vi "Test App Removing Process Triggers Broadcast.vi"(8 "error in (no error)":errorcluster, 11 "Rig Test in":refnum<class "Application Test.lvclass">) -> (0 "error out":errorcluster, 3 "Rig Test out":refnum<class "Application Test.lvclass">)   [LabVIEW 2020, in "Application Test.lvclass"]
uses:
  Application Test.lvclass
  C:/Program Files (x86)/National Instruments/LabVIEW 2020/vi.lib/Asteme/LUnit/Test Case.lvclass
  Framework/Process/Process.lvclass
  Framework/Process/Process.lvclass/Process.ctl
  Framework/Application/Application.lvclass/Application.ctl
  <vilib>/Asteme/LUnit/Test Case.lvclass/Test Case.ctl
  <vilib>/Asteme/LUnit/LUnit Assertion Result.lvclass/LUnit Assertion Result.ctl
  Framework/Application/Private/Add Process to Map.vi
  Framework/Application/Private/Start Idle Processes if Running.vi
  Framework/Process/Protected/Messaging/Enqueue Message.vi
  Framework/Process/Public/Lifecycle/Get Lifecycle State.vi
  Framework/Process/Protected/SubVIs/Set Context.vi
  Framework/Broadcast Event Helpers/Execution timer.vi
  <vilib>/Asteme/LUnit/Palette/Pass.vi
  <vilib>/Asteme/LUnit/Palette/Fail.vi
  <vilib>/Asteme/LUnit/Variant to string.vi
  <vilib>/Asteme/LUnit/Set Assertion Type.vi
  Framework/Process/Private/SubVIs/Wait for finish.vi
  Framework/Process/Private/SubVIs/Set Lifecycle State.vi
  <vilib>/Utility/error.llb/Clear Errors.vi
  Framework/Process/Public/Lifecycle/Leave Process Loop.vi
  <vilib>/Asteme/LUnit/Add test result.vi
  <vilib>/Asteme/LUnit/LUnit Write Passed.vi
  <vilib>/Asteme/LUnit/LUnit Get Test Case.vi
  <vilib>/Asteme/LUnit/Assertion Result/LUnit Get Test Name.vi
  <vilib>/Asteme/LUnit/LUnit Write Message.vi
  <vilib>/Asteme/LUnit/LUnit Write Description.vi
  <vilib>/Asteme/LUnit/LUnit Write Assertion Type.vi
  <vilib>/Asteme/LUnit/Read Test Case Name.vi
  Framework/Application/Application.lvclass
  C:/Users/anton/Documents/GitHub/Triarc-Framework/source/Framework/Process/Process.lvclass
  <vilib>/Utility/error.llb/Error Cluster From Error Code.vi
  Framework/Application/Private/Throw Error If Process Already in App.vi
  Framework/Application/Private/Update Context for Owned Processes.vi
  Framework/Broadcast Event Helpers/Dequeue Broadcast Message.vi
  <vilib>/Utility/Data Type/Get Type Information.vi
  <vilib>/Utility/LVClass/Get LV Class Name.vi
  <vilib>/Asteme/LUnit/LUnit Assertion Result.lvclass
  Framework/Broadcast Event Helpers/Broadcast Event Helpers.lvlib
  <vilib>/Asteme/LUnit/Test Case.lvclass
  C:/Users/anton/Documents/GitHub/Triarc-Framework/source/Framework/Base/Base.lvclass
  C:/Users/anton/Documents/GitHub/Triarc-Framework/source/Framework/Error Handler Interface/Error Handler Interface.lvclass
  C:/Users/anton/Documents/GitHub/Triarc-Framework/source/Framework/Logging/Logging.lvclass
  C:/Users/anton/Documents/GitHub/Triarc-Framework/source/Framework/Application/Application.lvclass
  C:/Users/anton/Documents/GitHub/Triarc-Framework/source/Framework/Async Handler/Async Handler.lvclass
  C:/Users/anton/Documents/GitHub/Triarc-Framework/source/Framework Test/Process Test/Process Test.lvclass
  C:/Users/anton/Documents/GitHub/Triarc-Framework/source/Framework Test/Base Class Test/Base Test.lvclass
  C:/Users/anton/Documents/GitHub/Triarc-Framework/source/Framework Test/Application Test/Application Test.lvclass
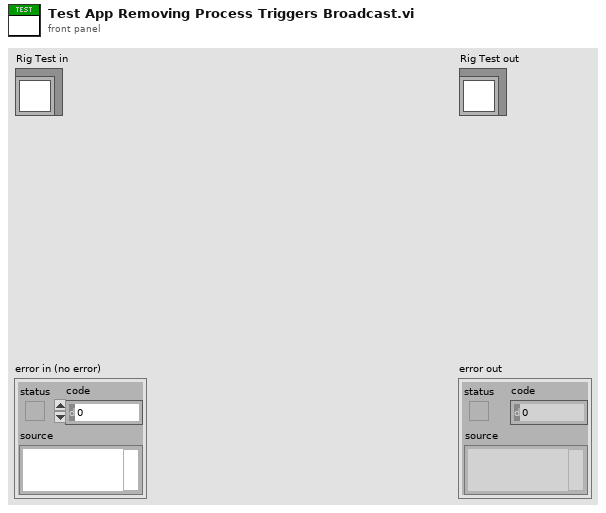
[diagram p1: front panel]
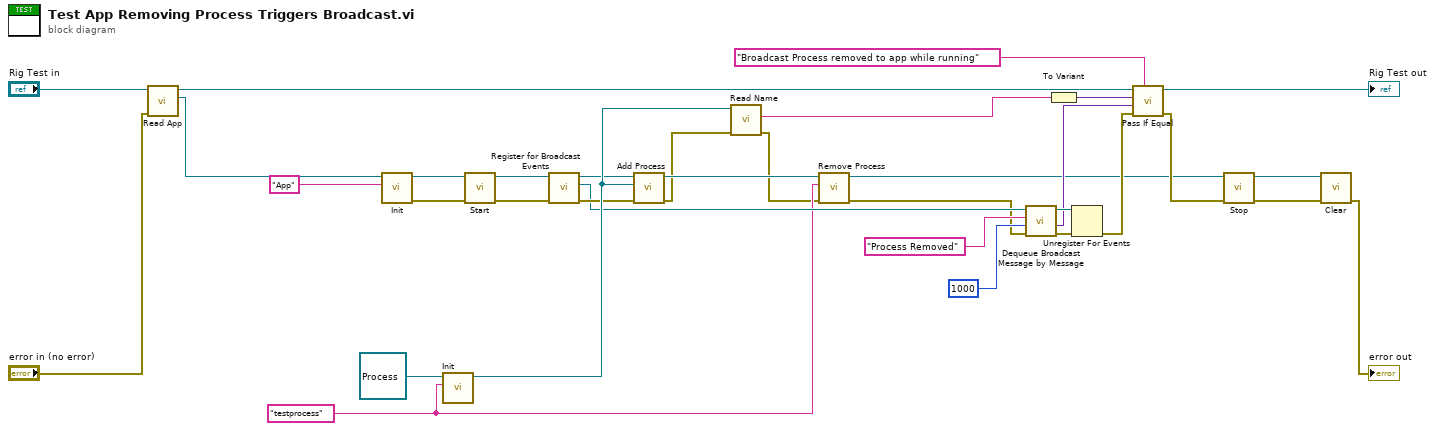
[diagram p0: block diagram]
diagram:
  w4 = "testprocess" ("Name")
  n1 = call "Read App.vi"("error in (no error)"="error in (no error)", "Application Test In"="Rig Test in") -> ("App out"=w33:refnum<class "Application.lvclass">, "Application Test Out"=w24:refnum<class "Application Test.lvclass">)  [unwired: 7 in, 1 out]
  n2 = call-dynamic "Init.vi"("Name"="App", "Process In"=w33) -> ("error out"=w25:errorcluster, "Process Out"=w26:refnum<class "Application.lvclass">)  [unwired: 8 in]
  n3 = call-dynamic "Init.vi"("Name"=w4, "Process In"=refnum<class "Process.lvclass"> refnum ("Process.lvclass")) -> ("Process Out"=w23:refnum<class "Process.lvclass">)  [unwired: 8 in, 1 out]
  n4 = call "Start.vi"("error in (no error)"=w25, "Process In"=w26) -> ("error out"=w27:errorcluster, "Process Out"=w17:refnum<class "Application.lvclass">)  [unwired: 7 in, 1 out]
  n5 = call "Register for Broadcast Events.vi"("error in (no error)"=w27, "Process In"=w17) -> ("error out"=w18:errorcluster, "Event Registration Refnum Out"=w14:refnum<event-registration>, "Process Out"=w16:refnum<class "Application.lvclass">)  [unwired: 7 in]
  n6 = call "Add Process.vi"("error in (no error)"=w18, "Process"=w23, "Rig In"=w16) -> ("error out"=w2:errorcluster, "Rig Out"=w6:refnum<class "Application.lvclass">)  [unwired: 7 in]
  n7 = call "Read Name.vi"("error in (no error)"=w2, "Process In"=w23) -> ("error out"=w3:errorcluster, "Qualified Name"=w15:string)  [unwired: 6 in, 2 out]
  n8 = call "Remove Process.vi"("error in (no error)"=w3, "Process Name"=w4, "Rig In"=w6) -> ("error out"=w1:errorcluster, "Rig Out"=w5:refnum<class "Application.lvclass">)  [unwired: 6 in, 1 out]
  n9 = call "Dequeue Broadcast Message by Message.vi"("error in (no error)"=w1, "Timeout (-1)"=1000, "Message"="Process Removed", "Event Registration Refnum"=w14) -> ("error out"=w13:errorcluster, "Message Data"=w10:variant, "Event Registration Refnum Out"=w11:refnum<event-registration>)  [unwired: 3 in, 2 out]
  n10 = To Variant(anything=w15) -> (Variant=w7:variant)
  n11 = Unregister For Events(event registration refnum=w11, error in=w13) -> (error out=w12:errorcluster)
  n12 = call <vilib>:"Pass If Equal.vi"("Description"="Broadcast Process removed to app while running", "error in (no error)"=w12, "Actual"=w10, "Expected"=w7, "Test Case In"=w24) -> ("error out"=w29:errorcluster, "Test Case Out"=→"Rig Test out":refnum<class "Application Test.lvclass">)  [unwired: 5 in]
  n13 = call "Stop.vi"("error in (no error)"=w29, "Process In"=w5) -> ("error out"=w21:errorcluster, "Process Out"=w20:refnum<class "Application.lvclass">)  [unwired: 7 in, 1 out]
  n14 = call-dynamic "Clear.vi"("error in (no error)"=w21, "Application In"=w20) -> ("error out"=→"error out":errorcluster)  [unwired: 9 in]
